vi "rd_var.vi"(8 "Index":i32=-1, 10 "var":T1 {"data" format="0x%08x"}) -> (0 "f32":sgl, 1 "i32":i32, 2 "u32":u32, 3 "bool":bool, 4 "String":string)   [LabVIEW 2014]
doc: "The VI sets the appropriate indicator in <B>bool</B>, <B>u32</B>, <B>i32</B> and <B>f32</B> depending on the type of <B>var</B>, returning default values in the rest of them."
uses:
  typedefs/var_t.ctl
  typedefs/val_type_t.ctl
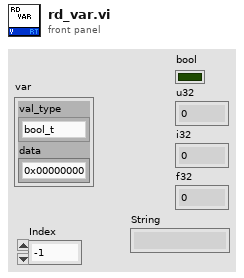
[diagram p1: front panel]
types:
  T1 = typedef "var_t.ctl" = cluster{"data":u32, "val_type":T2}
  T2 = typedef "val_type_t.ctl" = enum16{"bool_t", "i32_t", "u32_t", "f32_t"}
  T3 = typedef "LVDateTimeRec.ctl" = cluster{"fractional second":dbl, "second":i32, "minute":i32, "hour":i32, "day of month":i32, "month":i32, "year":i32, "day of week":i32, "day of year":i32, "DST":i32}
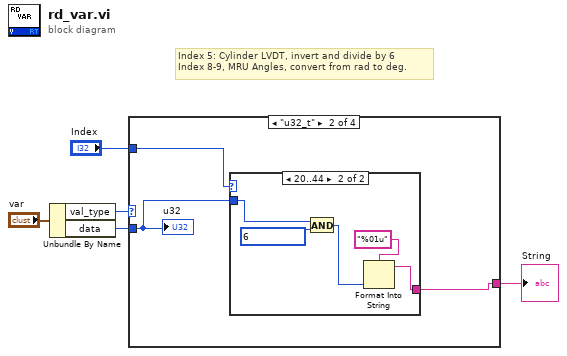
[diagram p0: block diagram]
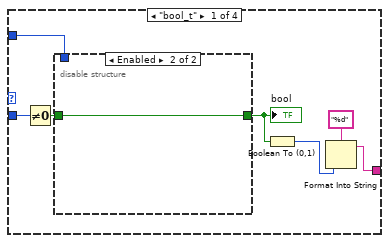
[diagram p2: hidden frame]
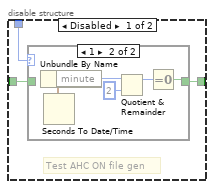
[diagram p3: hidden frame]
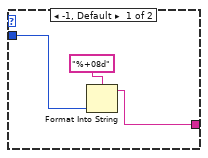
[diagram p5: hidden frame]
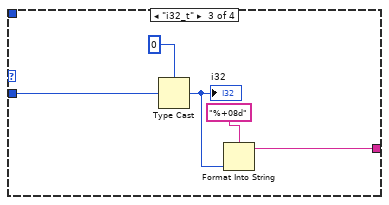
[diagram p6: hidden frame]
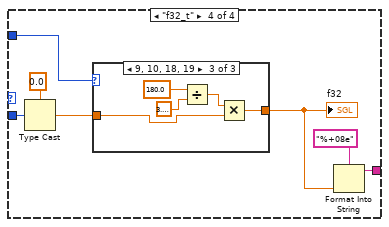
[diagram p7: hidden frame]
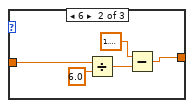
[diagram p9: hidden frame]
diagram:
  # "Index 5: Cylinder LVDT, invert and divide by 6\nIndex 8-9, MRU Angles, convert from rad to deg."
  n1 = Unbundle By Name("var") -> ("val_type"=w4:T2, "data"=w3:u32)
  n2 = case shown="\"u32_t\"" w4 {
    tunnel: w3 -> [w12 w24 w37 w44]
    tunnel: [w9 w23 w34 w43] -> w2
    tunnel: "Index" -> [w8 w25 _ w41]
    frame "bool_t" {
      n3 = Not Equal To 0?(x=w12) -> (x != 0?=w7:bool)
      n4 = disable-structure shown="Enabled" {
        disable-tunnel: w8 -> [w15 _]
        disable-tunnel: w7 -> [w14 w22]
        disable-tunnel: [w13 w22] -> w6
        frame Disabled {
          # "Test AHC ON file gen"
          n5 = case shown="1" w15 {
            tunnel: w14 -> [w16 _]
            tunnel: [w16 w17] -> w13
            frame 0, Default {
            }
            frame 1 {
              n6 = Seconds To Date/Time() -> (date time rec=w18:T3)  [unwired: 2 in]
              n7 = Unbundle By Name(w18) -> ("minute"=w19:i32)
              n8 = Quotient & Remainder(x=w19, y=2) -> (x-y*floor(x/y)=w21:i32)  [unwired: 1 out]
              n9 = Equal To 0?(x=w21) -> (x = 0?=w17:bool)
            }
          }
        }
        frame Enabled {
        }
      }
      "bool" <- w6
      n10 = Boolean To (0,1)(Boolean=w6) -> (0, 1=w10:i16)
      n11 = Format Into String(format string="%d", w10) -> (resulting string=w9:string)  [unwired: 2 in, 1 out]
    }
    frame "u32_t" {
      n12 = case shown="20..44" w25 {
        tunnel: w24 -> [w26 w32]
        tunnel: [w27 w29] -> w23
        frame -1, Default {
          n13 = Format Into String(format string="%+08d", w26) -> (resulting string=w27:string)  [unwired: 2 in, 1 out]
        }
        frame 20..44 {
          n14 = And(x=w32, y=u32 6) -> (x .and. y?=w30:u32)
          n15 = Format Into String(format string="%01u", w30) -> (resulting string=w29:string)  [unwired: 2 in, 1 out]
        }
      }
      "u32" <- w24
    }
    frame "i32_t" {
      n16 = Type Cast(type=0, x=w37) -> (*(type *) &x=w35:i32)
      "i32" <- w35
      n17 = Format Into String(format string="%+08d", w35) -> (resulting string=w34:string)  [unwired: 2 in, 1 out]
    }
    frame "f32_t" {
      n18 = Type Cast(type=sgl 0.0, x=w44) -> (*(type *) &x=w40:sgl)
      n19 = case shown="9, 10, 18, 19" w41 {
        tunnel: w40 -> [w46 w51 w52]
        tunnel: [w46 w47 w54] -> w39
        frame -1, Default {
        }
        frame 6 {
          n20 = Divide(x=w51, y=sgl 6.0) -> (x/y=w49:sgl)
          n21 = Subtract(x=sgl 1.1, y=w49) -> (x-y=w47:sgl)
        }
        frame 9, 10, 18, 19 {
          n22 = Divide(x=sgl 180.0, y=sgl 3.1415927) -> (x/y=w53:sgl)
          n23 = Multiply(x=w53, y=w52) -> (x*y=w54:sgl)
        }
      }
      "f32" <- w39
      n24 = Format Into String(format string="%+08e", w39) -> (resulting string=w43:string)  [unwired: 2 in, 1 out]
    }
  }
  "String" <- w2
